vi "Localization Demo.vi"() -> ()   [LabVIEW 2017]
uses:
  Private/RegisterVI.vi
  <vilib>/Platform/browser.llb/Open URL in Default Browser (string).vi
  API/JKI Simple Localization.lvlib
panel:
  in  "Language ListBox":i32(listbox) caption="Language"
  in  "Target Language (optional)":string
  out "Translated Phrase":string
  in  "Translate Me":string
  out "Data.Display":dbl(graph) caption="Incoming Data"
  out "Error":bool
  in  "CustomControl.Increment":bool caption="Increment"
  out "Count":dbl
  in  "Exit":bool
  # "Translate Phrase"
  # "Key: \"Error\" (Label)\nDisplay Name: \"ERROR\" (Caption)"
  # "Key: \"CustomControl.Increment\" (Label)\nDisplay Name: Increment (Caption)\nBoolean Text (True): Okay\nBoolean Text (False): +1"
  # "Key: \"Language Ring\" (Label)\nDisplay Name: \"Language\" (Caption)"
  # "Key: \"Count\" (Label)\nDisplay Name: \"Count\" (Caption)"
  # "Key: \"Data.Display\" (Label)\nDisplay Name: \"Incoming Data\" (Caption)\nX Axis: Time (sec)\nY Axis: Voltage (V)"
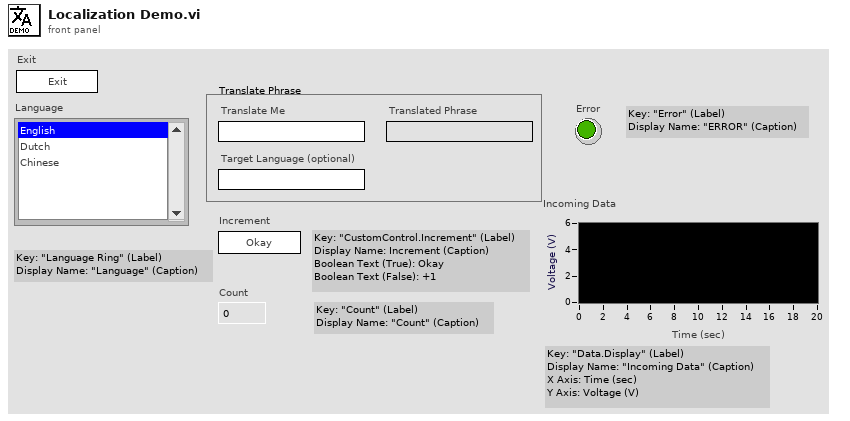
[diagram p1: front panel]
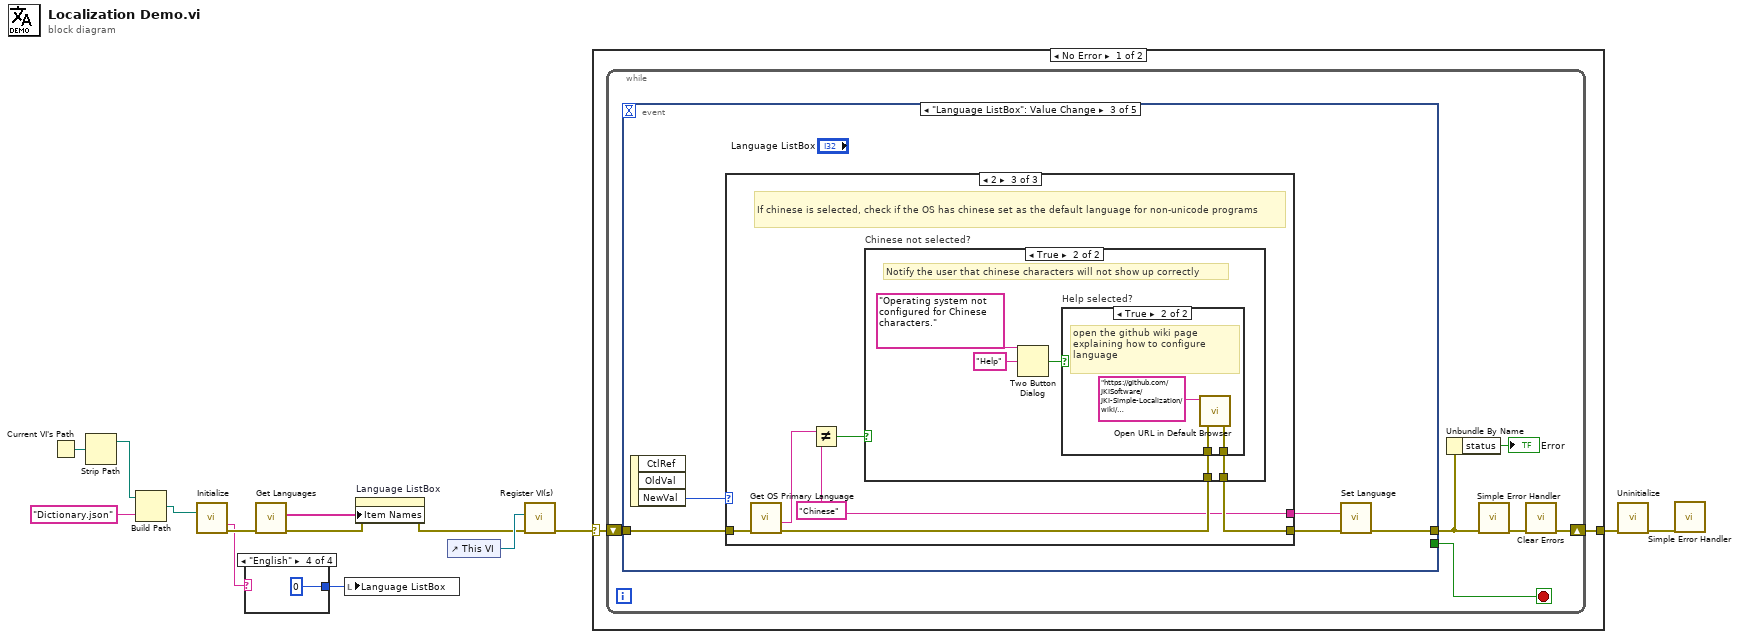
[diagram p0: block diagram]
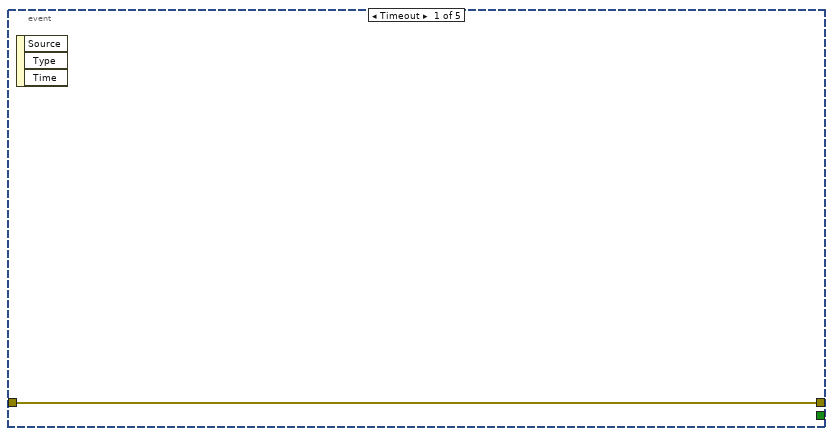
[diagram p2: hidden frame]
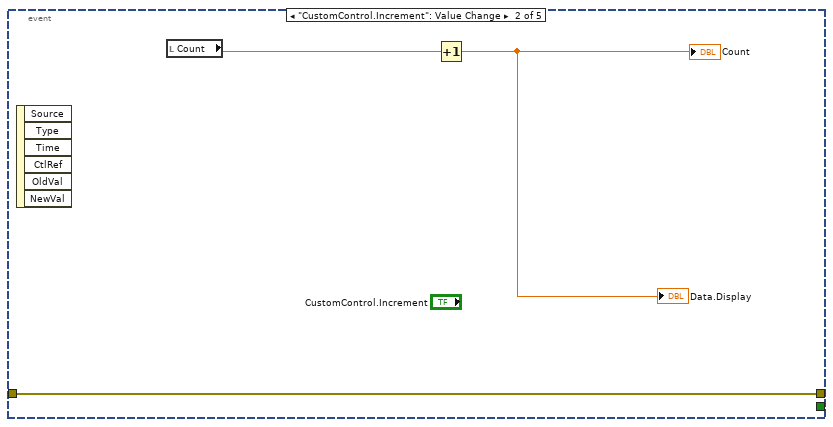
[diagram p3: hidden frame]
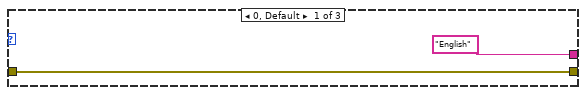
[diagram p4: hidden frame]
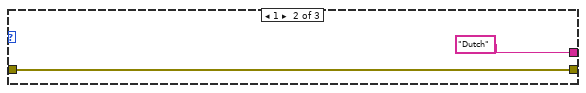
[diagram p5: hidden frame]
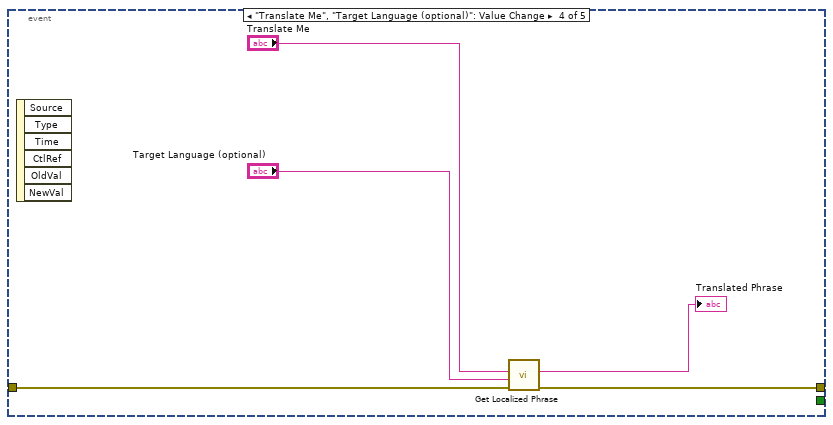
[diagram p8: hidden frame]
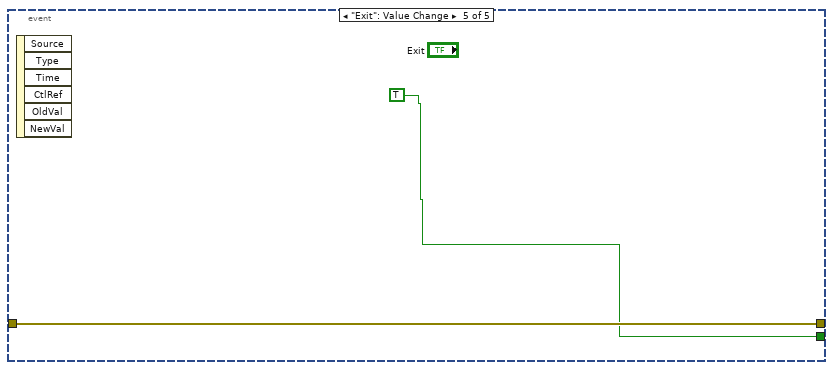
[diagram p9: hidden frame]
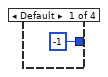
[diagram p11: hidden frame]
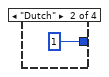
[diagram p12: hidden frame]
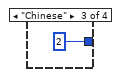
[diagram p13: hidden frame]
diagram:
  n1 = Current VI's Path() -> (path=w2:path)
  n2 = Strip Path(path=w2) -> (stripped path=w1:path)  [unwired: 1 out]
  n3 = Build Path(base path=w1, name or relative path="Dictionary.json") -> (appended path=w13:path)
  n4 = call "Initialize.vi"("Dictionary File Path"=w13) -> ("Current Language"=w5:string, "error out"=w8:errorcluster)  [unwired: 11 in, 2 out]
  n5 = case shown="\"English\"" w5 {
    tunnel: [-1 ("Language ListBox") 1 ("Language ListBox") 2 ("Language ListBox") 0 ("Language ListBox")] -> w6
    frame Default {
    }
    frame "Dutch" {
    }
    frame "Chinese" {
    }
    frame "English" {
    }
  }
  n6 = call "Get Languages.vi"("error in"=w8) -> ("error out"=w10:errorcluster, "Languages"=w11:string[])  [unwired: 9 in]
  n7 = local write "Language ListBox"(w6) -> ()
  n8 = property on="Language ListBox" class="LstBox (strict)"(error in=w10, "Item Names"=w11) -> (error out=w7:errorcluster)  [unwired: 1 in, 1 out]
  n9 = control-ref of="This VI"() -> (w12:refnum<vi>)
  n10 = call-poly "Register VI(s).vi"("error in"=w7, "VI Ref"=w12) -> ("error out"=w4:errorcluster)  [unwired: 8 in, 1 out]
  n11 = case shown="No Error" w4 {
    selector: w4 -> [w19 w63]
    tunnel: [w20 w63] -> w9
    frame No Error {
      n12 = while {
        shift-right: [w23] -> w20
        shift-left: w19 -> [w25]
        stop <- w26 stop-if-true
        n13 = event shown="[2] \"Language ListBox\": Value Change" {
          selector: _ -> [_ _ _ _ _]
          dyn-events: _ -> [_ _ _ _ _]
          timeout: _ -> [_ _ _ _ _]
          tunnel: [_ _ _ _ TRUE ("Exit")] -> w26
          tunnel: [w27 w28 w34 w59 w62] -> w21
          tunnel: w25 -> [w27 w28 w32 w60 w62]
          event Timeout {
            n14 = event-data() -> ()  [unwired: 1 in, 3 out]
          }
          event "CustomControl.Increment": Value Change {
            n15 = event-data() -> ()  [unwired: 1 in, 6 out]
            n16 = local read "Count"() -> (w30:dbl)
            n17 = Increment(x=w30) -> (x+1=→"Count" →"Data.Display":dbl)
          }
          event "Language ListBox": Value Change {
            n18 = event-data() -> ("NewVal"=w35:i32)  [unwired: 1 in, 2 out]
            n19 = case shown="2" w35 {
              tunnel: ["English" ("name or relative path") "Dutch" ("name or relative path") w40] -> w33
              tunnel: w32 -> [w36 w38 w45]
              tunnel: [w36 w38 w41] -> w31
              frame 0, Default {
              }
              frame 1 {
              }
              frame 2 {
                w40 = "Chinese" ("name or relative path")
                # "If chinese is selected, check if the OS has chinese set as the default language for non-unicode programs"
                n20 = call "Get OS Primary Language.vi"("error in"=w45) -> ("error out"=w42:errorcluster, "OS Primary Language"=w44:string)  [unwired: 9 in]
                n21 = Not Equal?(x=w44, y=w40) -> (x != y?=w43:bool)
                n22 = case "Chinese not selected?" shown="True" w43 {
                  tunnel: w42 -> [w46 w48]
                  tunnel: [w46 w47] -> w41
                  frame False {
                    # "Chinese characters will show up correctly"
                  }
                  frame True {
                    # "Notify the user that chinese characters will not show up correctly"
                    n23 = Two Button Dialog(message="Operating system not configured for Chinese characters.", 2:"Help" ("T button name (\"OK\")")) -> (T button?=w49:bool)  [unwired: 1 in]
                    n24 = case "Help selected?" shown="True" w49 {
                      tunnel: w48 -> [w52 w54]
                      tunnel: [w52 w53] -> w47
                      frame False {
                      }
                      frame True {
                        # "open the github wiki page explaining how to configure language"
                        n25 = call-poly <vilib>:"Open URL in Default Browser.vi"("error in (no error)"=w54, "URL"="https://github.com/JKISoftware/JKI-Simple-Localization/wiki/Configuring-Windows-Language-(System-Locale)") -> ("error out"=w53:errorcluster)  [unwired: 4 in, 1 out]
                      }
                    }
                  }
                }
              }
            }
            n26 = call "Set Language.vi"("error in"=w31, "Target Language (current lang)"=w33) -> ("error out"=w34:errorcluster)  [unwired: 8 in, 1 out]
          }
          event "Translate Me", "Target Language (optional)": Value Change {
            n27 = event-data() -> ()  [unwired: 1 in, 6 out]
            n28 = call "Get Localized Phrase.vi"("error in"=w60, "Target Language (current lang)"="Target Language (optional)", "Key"="Translate Me") -> ("error out"=w59:errorcluster, "Translated Phrase"=→"Translated Phrase":string)  [unwired: 7 in]
          }
          event "Exit": Value Change {
            n29 = event-data() -> ()  [unwired: 1 in, 6 out]
          }
        }
        n30 = Unbundle By Name(w21) -> ("status"=→"Error":bool)
        n31 = call <vilib>:"Simple Error Handler.vi"("error in (no error)"=w21) -> ("error out"=w22:errorcluster)  [unwired: 4 in, 4 out]
        n32 = call <vilib>:"Clear Errors.vi"("error in (no error)"=w22) -> ("error out"=w23:errorcluster)  [unwired: 5 in, 1 out]
      }
    }
    frame Error {
    }
  }
  n33 = call "Uninitialize.vi"("error in"=w9) -> ("error out"=w3:errorcluster)  [unwired: 10 in]
  n34 = call <vilib>:"Simple Error Handler.vi"("error in (no error)"=w3) -> ()  [unwired: 4 in, 5 out]
